vi "Recognition.Leitura.vi"(8 "error in (no error)":errorcluster) -> (0 "error out":errorcluster, 2 "SemSenha":bool, 3 "Senha":i32[](array[numeric]))   [LabVIEW 2019]
uses:
  <vilib>/Utility/xml.llb/Read From XML File(string).vi
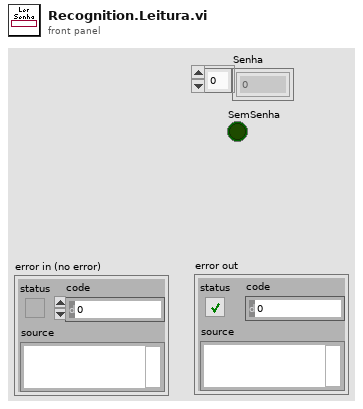
[diagram p1: front panel]
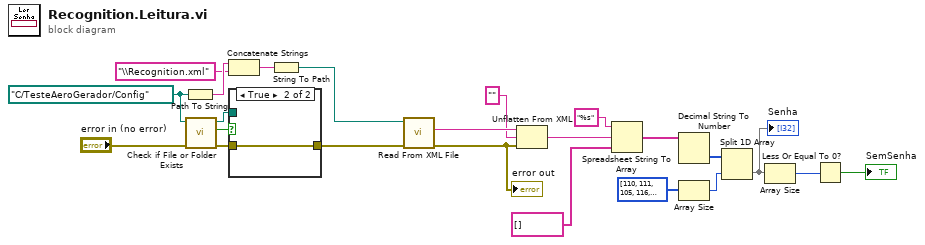
[diagram p0: block diagram]
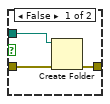
[diagram p2: hidden frame]
diagram:
  w20 = path "C:/TesteAeroGerador/Config" ("XML File Path")
  n1 = Path To String(path=w20) -> (string=w19:string)
  n2 = call <vilib>:"Check if File or Folder Exists.vi"("error in (no error)"="error in (no error)", "path"=w20) -> ("error out"=w22:errorcluster, "file or folder exists?"=w23:bool, "dup path"=w16:path)  [unwired: 7 in]
  n3 = Concatenate Strings(w19, "\\Recognition.xml") -> (w17:string)
  n4 = case shown="True" w23 {
    tunnel: w16 -> [w26 _]
    tunnel: w22 -> [w25 w27]
    tunnel: [w24 w27] -> w15
    frame False {
      n5 = Create Folder(path (use dialog)=w26, error in=w25) -> (error out=w24:errorcluster)  [unwired: 1 in, 2 out]
    }
    frame True {
    }
  }
  n6 = String To Path(string=w17) -> (path=w14:path)
  n7 = call-poly <vilib>:"Read From XML File.vi"("error in (no error)"=w15, "XML File Path"=w14) -> ("error out"=w12:errorcluster, "XML Elements"=w13:string)  [unwired: 7 in, 1 out]
  "error out" <- w12
  n8 = Unflatten From XML(xml string=w13, type="", error in (no error)=w12) -> (value=w8:string)  [unwired: 1 out]
  n9 = Spreadsheet String To Array(format string="%s", spreadsheet string=w8, array type (2D Dbl)=string[] []) -> (array=w7:string[])  [unwired: 1 in]
  n10 = Decimal String To Number(string=w7) -> (number=w4:i32[])  [unwired: 2 in, 1 out]
  n11 = Array Size(array=u8[] [110, 111, 105, 116, 105, 110, 103, 111, 99, 101, 82] ("unsigned byte array")) -> (size(s)=w5:i32)
  n12 = Split 1D Array(array=w4, index=w5) -> (second subarray=w3:i32[])  [unwired: 1 out]
  "Senha" <- w3
  n13 = Array Size(array=w3) -> (size(s)=w2:i32)
  n14 = Less Or Equal To 0?(x=w2) -> (x <= 0?=→"SemSenha":bool)
